vi "Display status FGV.vi"(6 "Action":T1, 8 "error in":errorcluster, 10 "Input":string) -> (0 "error out":errorcluster, 2 "Display":string)   [LabVIEW 2015]
uses:
  FGV action.ctl
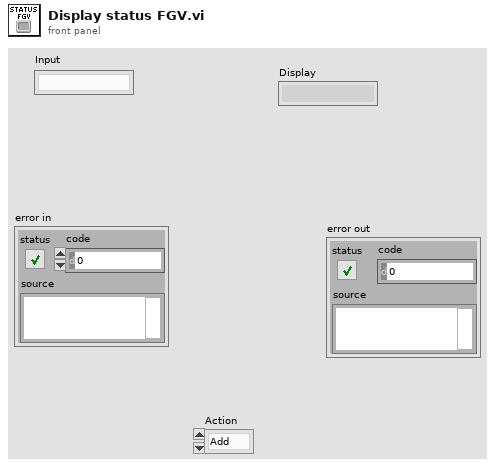
[diagram p1: front panel]
types:
  T1 = typedef "FGV action.ctl" = enum16{"Add", "Get", "Clear"}
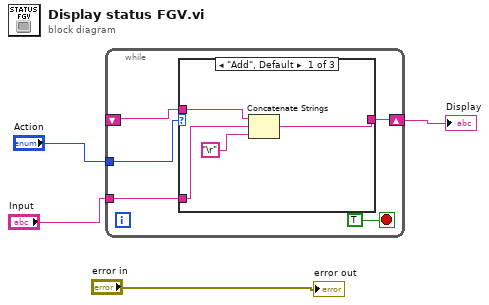
[diagram p0: block diagram]
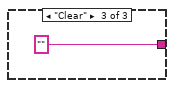
[diagram p3: hidden frame]
diagram:
  n1 = while {
    shift-right: [w7] -> w2
    shift-left: _ -> [w6]
    tunnel: "Action" -> [w8]
    tunnel: "Input" -> [w5]
    stop <- TRUE stop-if-true
    n2 = case shown="\"Add\", Default" w8 {
      tunnel: [w11 w14 "" ("String")] -> w7
      tunnel: w6 -> [w13 w14 _]
      tunnel: w5 -> [w12 _ _]
      frame "Add", Default {
        n3 = Concatenate Strings(w13, w12, "\r") -> (w11:string)
      }
      frame "Get" {
      }
      frame "Clear" {
      }
    }
  }
  "Display" <- w2
  "error out" <- "error in"
